vi "Write Indent String.vi"(8 "error in (no error)":errorcluster, 10 "Indent String":string="    ", 11 "JSON Serializer in":refnum<class "JSON Serializer.lvclass">) -> (0 "error out":errorcluster, 3 "JSON Serializer out":refnum<class "JSON Serializer.lvclass">)   [LabVIEW 2019, in "JKI JSON Serialization.lvlib" / "JSON Serializer.lvclass"]
doc: "Specifies the indent string used for pretty-print.\n\nJKI JSON 1.1.10.37\nTomi Maila - JKI\nCopyright (c) 2017, JKI"
uses:
  JSON Serializer.lvclass
  JSON Serializer.lvclass/JSON Serializer.ctl
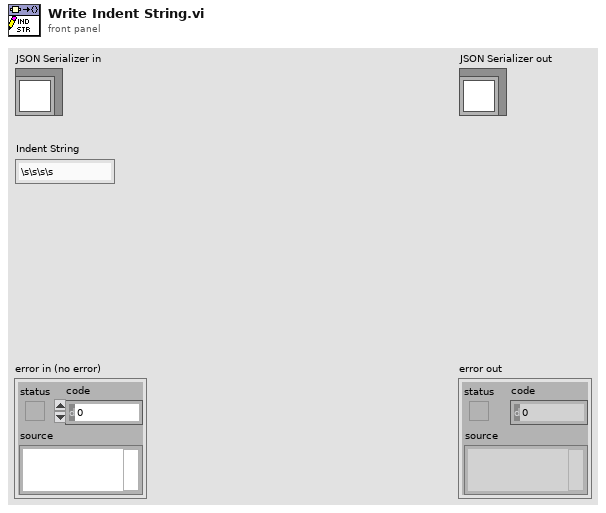
[diagram p1: front panel]
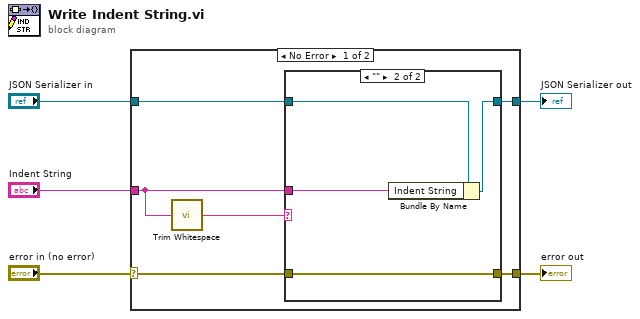
[diagram p0: block diagram]
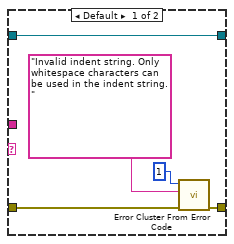
[diagram p2: hidden frame]
diagram:
  n1 = case shown="No Error" "error in (no error)" {
    selector: "error in (no error)" -> [w7 w21]
    tunnel: [w6 w21] -> w4
    tunnel: [w10 w22] -> w2
    tunnel: "JSON Serializer in" -> [w11 w22]
    tunnel: "Indent String" -> [w8 _]
    frame No Error {
      n2 = call <vilib>:"Trim Whitespace.vi"("string"=w8) -> ("trimmed string"=w9:string)  [unwired: 1 in]
      n3 = case shown="\"\"" w9 {
        tunnel: w11 -> [w16 w20]
        tunnel: [w16 w19] -> w10
        tunnel: w8 -> [_ w18]
        tunnel: w7 -> [w14 w17]
        tunnel: [w15 w17] -> w6
        frame Default {
          n4 = call <vilib>:"Error Cluster From Error Code.vi"("error in (no error)"=w14, "error message (\"\")"="Invalid indent string. Only whitespace characters can be used in the indent string." ("error message (\"\")"), "error code (0)"=1) -> ("error out"=w15:errorcluster)  [unwired: 6 in]
        }
        frame "" {
          n5 = Bundle By Name(cluster=w20, "Indent String"=w18) -> (w19:refnum<class "JSON Serializer.lvclass">)
        }
      }
    }
    frame Error {
    }
  }
  "error out" <- w4
  "JSON Serializer out" <- w2
